vi "SelectMixtures.vi"(8 "Max Number of Odors":u16=10, 9 "Concentrations":string[](array[string]), 10 "Odors":string[](array[string])) -> (2 "Canceled?":bool, 3 "Odor Mixtures":bool[](array[boolean]))   [LabVIEW 2016]
panel:
  in  "OK Button":bool
  in  "Cancel Button":bool
  in  "cluster 2":T1
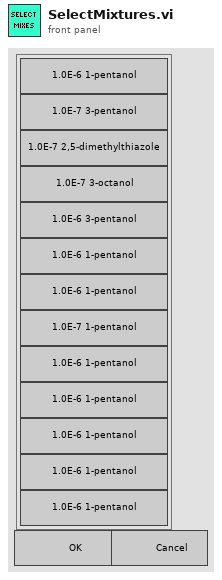
[diagram p1: front panel]
types:
  T1 = cluster{"Odors[0]":bool, "Odors[0] 2":bool, "Odors[0] 3":bool, "Odors[0] 4":bool, "Odors[0] 5":bool, "Odors[0] 6":bool, "Odors[0] 7":bool, "Odors[0] 8":bool, "Odors[0] 9":bool, "Odors[0] 10":bool, "Odors[0] 11":bool, "Odors[0] 12":bool, "Odors[0] 13":bool}
  T2 = cluster{"[0]":bool, "[1]":bool, "[2]":bool, "[3]":bool, "[4]":bool, "[5]":bool, "[6]":bool, "[7]":bool, "[8]":bool, "[9]":bool, "[10]":bool, "[11]":bool, "[12]":bool}
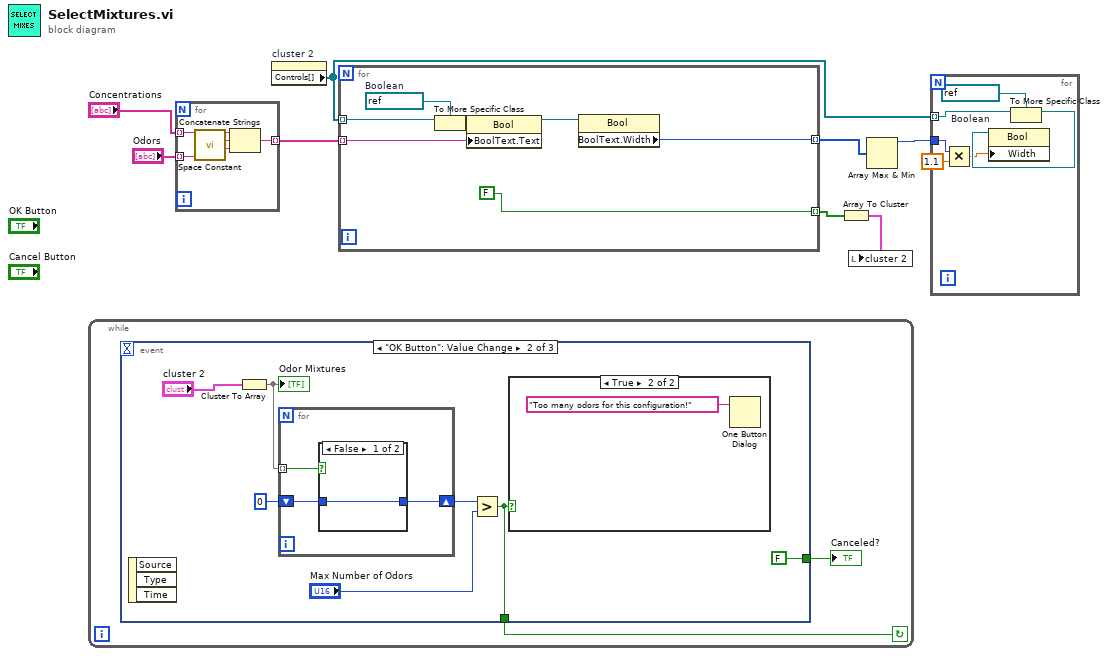
[diagram p0: block diagram]
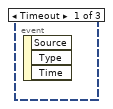
[diagram p2: hidden frame]
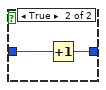
[diagram p3: hidden frame]
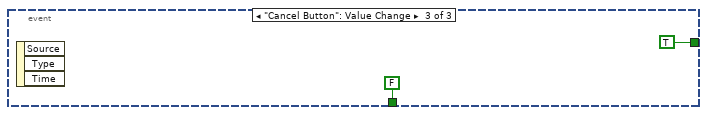
[diagram p5: hidden frame]
diagram:
  n1 = while {
    stop <- w9 continue-if-true
    n2 = event shown="[1] \"OK Button\": Value Change" {
      selector: _ -> [_ _ _]
      dyn-events: _ -> [_ _ _]
      timeout: _ -> [_ _ _]
      tunnel: [_ FALSE TRUE] -> w10
      tunnel: [_ w11 FALSE] -> w9
      event Timeout {
        n3 = event-data() -> ()  [unwired: 1 in, 3 out]
      }
      event "OK Button": Value Change {
        n4 = event-data() -> ()  [unwired: 1 in, 3 out]
        n5 = Cluster To Array(cluster="cluster 2") -> (array=w15:bool[])
        "Odor Mixtures" <- w15
        n6 = for {
          tunnel: w15 -> [w20] mode=indexing
          shift-right: [w18] -> w13
          shift-left: 0 -> [w19]
          n7 = case shown="False" w20 {
            tunnel: w19 -> [w21 w23]
            tunnel: [w21 w22] -> w18
            frame False {
            }
            frame True {
              n8 = Increment(x=w23) -> (x+1=w22:i32)
            }
          }
        }
        n9 = Greater?(x=w13, y="Max Number of Odors") -> (0:w11:bool)
        n10 = case shown="True" w11 {
          frame False {
          }
          frame True {
            n11 = One Button Dialog(message="Too many odors for this configuration!") -> ()  [unwired: 1 in, 1 out]
          }
        }
      }
      event "Cancel Button": Value Change {
        n12 = event-data() -> ()  [unwired: 1 in, 3 out]
      }
    }
    "Canceled?" <- w10
  }
  n13 = for {
    tunnel: "Concentrations" -> [w30] mode=indexing
    tunnel: "Odors" -> [w28] mode=indexing
    tunnel: [w27] -> w6 mode=indexing
    n14 = call <vilib>:"Space Constant.vi"() -> ("String"=w29:string)
    n15 = Concatenate Strings(w30, w29, w28) -> (w27:string)
  }
  n16 = property on="cluster 2" class="Clust (strict)"() -> ("Controls[]"=w4:refnum<vi>[])  [unwired: 2 in, 2 out]
  n17 = for {
    tunnel: w4 -> [w36] mode=indexing
    tunnel: w6 -> [w37] mode=indexing
    tunnel: [w32] -> w5 mode=indexing
    tunnel: [FALSE] -> w2 mode=indexing
    w35 = refnum<vi> refnum  # Boolean
    n18 = To More Specific Class(target class=w35, reference=w36) -> (specific class reference=w34:refnum<vi>)  [unwired: 1 in, 1 out]
    n19 = property class="Bool"(reference=w34, "BoolText.Text"=w37) -> (reference out=w33:refnum<vi>)  [unwired: 1 in, 1 out]
    n20 = property class="Bool"(reference=w33) -> ("BoolText.Width"=w32:u32)  [unwired: 1 in, 2 out]
  }
  n21 = Array To Cluster(array=w2) -> (cluster=w1:T2)
  n22 = local write "cluster 2"(w1) -> ()
  n23 = Array Max & Min(array=w5) -> (max value=w3:u32)  [unwired: 3 out]
  n24 = for {
    tunnel: w4 -> [w43] mode=indexing
    tunnel: w3 -> [w40]
    w42 = refnum<vi> refnum  # Boolean
    n25 = Multiply(x=w40, y=1.1) -> (x*y=w38:dbl)
    n26 = To More Specific Class(target class=w42, reference=w43) -> (specific class reference=w41:refnum<vi>)  [unwired: 1 in, 1 out]
    n27 = property class="Bool"(reference=w41, "Width"=w38) -> ()  [unwired: 1 in, 2 out]
  }
